vi "Int8Array Create (Dimensions).vi"(8 "error in (no error)":errorcluster, 10 "Array dimensions":i32[](array[numeric]), 11 "I8 array in":i8[](array[numeric])) -> (0 "error out":errorcluster, 3 "Int8Array DVR out":refnum<data-value>)   [LabVIEW 2012, in "MDSplus.lvlib"]
uses:
  <vilib>/MDSplus/Library/MDSplus.lvlib
  <vilib>/MDSplus/Classes/Data_Class/Array_Class/Int8Array_Class/Int8Array.lvclass
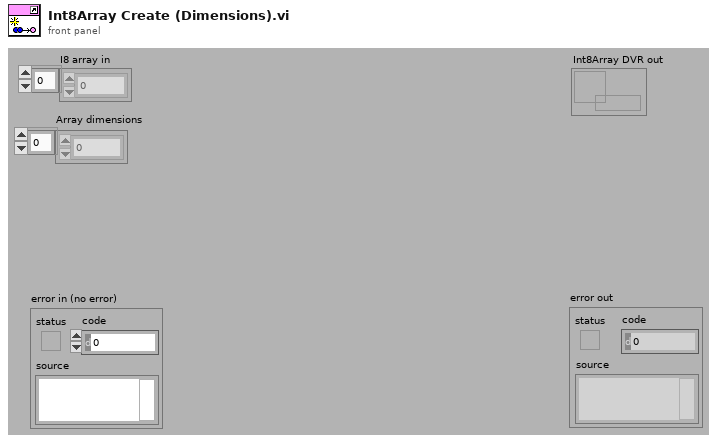
[diagram p1: front panel]
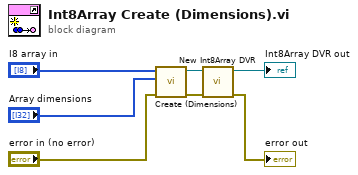
[diagram p0: block diagram]
diagram:
  n1 = call <vilib>:"Create (Dimensions).vi"("error in (no error)"="error in (no error)", "Dimensions"="Array dimensions", "I8 array in"="I8 array in") -> ("error out"=w4:errorcluster, "Int8Array out"=w5:refnum<class "Int8Array.lvclass">)  [unwired: 7 in]
  n2 = call <vilib>:"New Int8Array DVR.vi"("error in (no error)"=w4, "Int8Array in"=w5) -> ("error out"=→"error out":errorcluster, "Int8Array DVR out"=→"Int8Array DVR out":refnum<data-value>)  [unwired: 8 in]
